vi "findStageIndexes.vi"(8 "error in (no error)":errorcluster, 10 "index":i32, 11 "ScriptEventList in":refnum<class "ScriptEventList.lvclass">) -> (0 "error out":errorcluster, 1 "noneFound":bool, 2 "indexArray":i32[](array[numeric]), 3 "ScriptEventList out":refnum<class "ScriptEventList.lvclass">)   [LabVIEW 2009, in "Tools.lvlib" / "Scripting.lvlib" / "ScriptEventList.lvclass"]
uses:
  ScriptEventList.lvclass
  ScriptEventList.lvclass/ScriptEventList.ctl
  ScriptEvent.lvclass
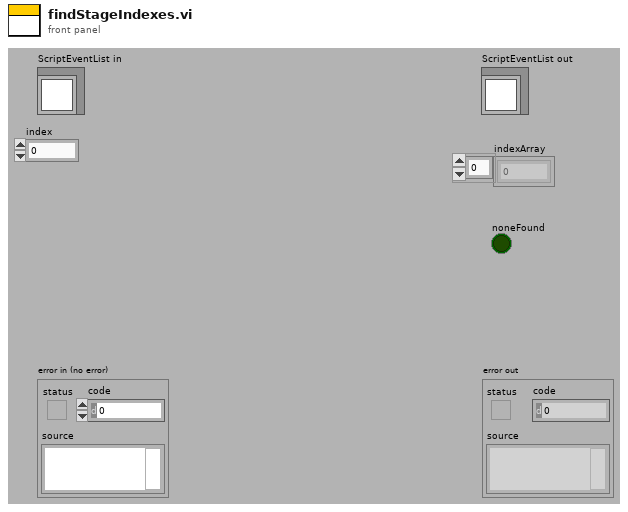
[diagram p1: front panel]
types:
  T1 = enum16{"Initialise", "MOT", "Molasses", "Optical Pumping", "Magnetic Trap", "RF Cooling", "Manipulation", "Switch Off", "Absorption Imaging", "Fluorscence Imaging", "Shut Down"}
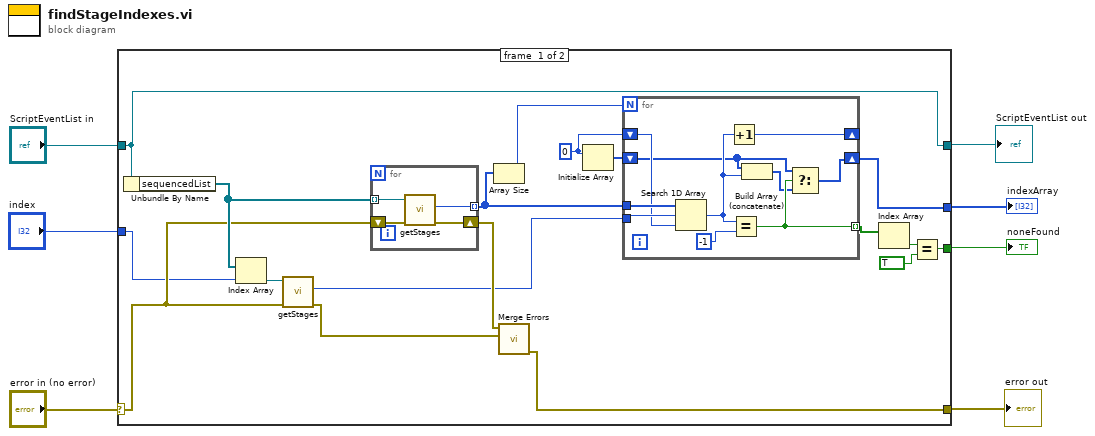
[diagram p0: block diagram]
diagram:
  n1 = case shown="No Error" "error in (no error)" {
    selector: "error in (no error)" -> [w22 w41]
    tunnel: [w17 w41] -> w6
    tunnel: [w25 w40] -> w4
    tunnel: "ScriptEventList in" -> [w25 w40]
    tunnel: "index" -> [w9 _]
    tunnel: [w12 _] -> w1
    tunnel: [w13 _] -> w2
    frame #0 {
      w8 = 0
      n2 = Unbundle By Name(w25) -> ("sequencedList"=w23:refnum<class "ScriptEvent.lvclass">[])
      n3 = Index Array(array=w23, index=w9) -> (element=w24:refnum<class "ScriptEvent.lvclass">)
      n4 = call "getStages.vi"("error in (no error)"=w22, "ScriptEvent.lvclass in"=w24) -> ("error out"=w18:errorcluster, "Stage"=w10:T1)  [unwired: 7 in, 1 out]
      n5 = for {
        tunnel: w23 -> [w39] mode=indexing
        tunnel: [w38] -> w20 mode=indexing
        shift-right: [w36] -> w19
        shift-left: w22 -> [w37]
        n6 = call "getStages.vi"("error in (no error)"=w37, "ScriptEvent.lvclass in"=w39) -> ("error out"=w36:errorcluster, "Stage"=w38:T1)  [unwired: 7 in, 1 out]
      }
      n7 = Array Size(array=w20) -> (size(s)=w21:i32)
      n8 = call <vilib>:"Merge Errors.vi"("error in 2 (no error)"=w18, "error in 1 (no error)"=w19) -> ("error out"=w17:errorcluster)  [unwired: 5 in]
      n9 = Initialize Array(w8) -> (w11:i32[])  [unwired: 1 in]
      n10 = for {
        N: w21 -> [_]
        tunnel: w20 -> [w35]
        tunnel: w10 -> [w34]
        shift-right: [w31] -> _
        shift-left: w8 -> [w32]
        tunnel: [w30] -> w15 mode=indexing
        shift-right: [w27] -> w12
        shift-left: w11 -> [w26]
        n11 = Search 1D Array(1D array=w35, element=w34, start index (0)=w32) -> (index of element=w29:i32)
        n12 = Increment(x=w29) -> (x+1=w31:i32)
        n13 = Equal?(x=w29, y=-1) -> (x = y?=w30:bool)
        n14 = Build Array (concatenate)(w26, w29) -> (w28:i32[])
        n15 = Select(t=w26, s=w30, f=w28) -> (s? t:f=w27:i32[])
      }
      n16 = Index Array(array=w15) -> (element=w16:bool)  [unwired: 1 in]
      n17 = Equal?(x=w16, y=TRUE) -> (x = y?=w13:bool)
    }
    frame #1 {
    }
  }
  "error out" <- w6
  "ScriptEventList out" <- w4
  "noneFound" <- w2
  "indexArray" <- w1
